vi "loadChannel.vi"(6 "xmlPath":string, 8 "error in (no error)":errorcluster, 9 "device.lvclass":refnum<class "device.lvclass">, 10 "NativeXML in":refnum<class "NativeXML.lvclass">, 11 "deviceDataBase in":refnum<class "deviceDataBase.lvclass">) -> (0 "error out":errorcluster, 1 "device.lvclass out":refnum<class "device.lvclass">, 2 "Channel.lvclass":refnum<class "Channel.lvclass">, 3 "deviceDataBase out":refnum<class "deviceDataBase.lvclass">)   [LabVIEW 2009, in "Tools.lvlib" / "DatabaseHelpers.lvlib" / "deviceDataBase.lvclass"]
uses:
  deviceDataBase.lvclass
  NativeXML/NativeXML.lvclass
  Database Objects/device/device.lvclass
  Database Objects/Channel/Channel.lvclass
  Database Objects/Channel/DigitalChannel/DigitalChannel.lvclass
  Database Objects/Channel/RfOutputChannel/RfOutputChannel.lvclass
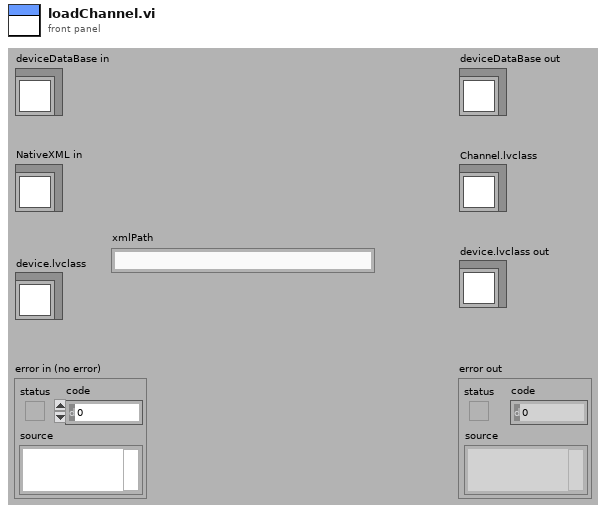
[diagram p1: front panel]
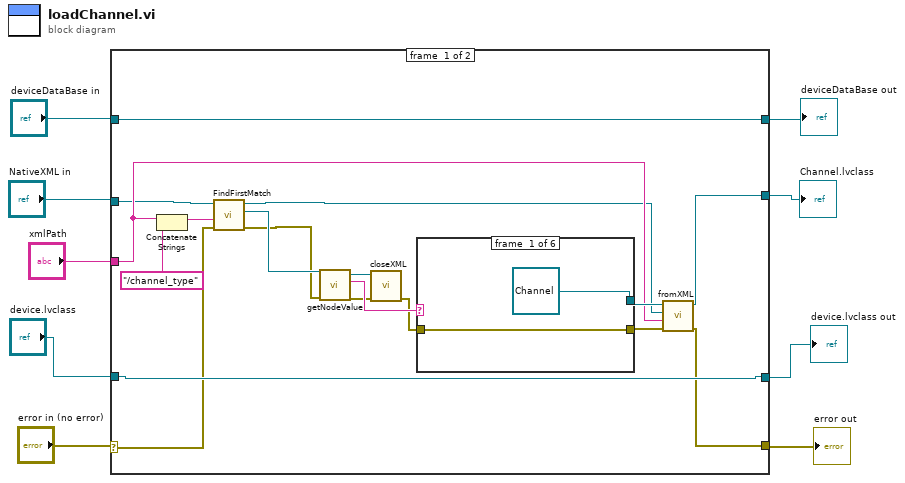
[diagram p0: block diagram]
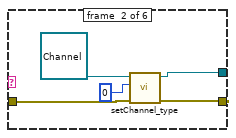
[diagram p2: hidden frame]
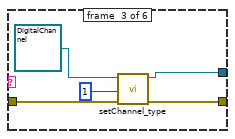
[diagram p3: hidden frame]
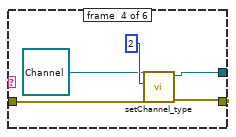
[diagram p4: hidden frame]
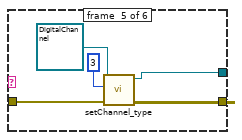
[diagram p5: hidden frame]
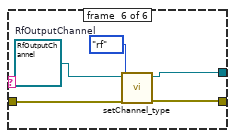
[diagram p6: hidden frame]
diagram:
  n1 = case shown="No Error" "error in (no error)" {
    selector: "error in (no error)" -> [w11 w56]
    tunnel: [w23 w56] -> w8
    tunnel: [w22 w55] -> w6
    tunnel: "deviceDataBase in" -> [w22 w55]
    tunnel: "device.lvclass" -> [w27 _]
    tunnel: "NativeXML in" -> [w14 _]
    tunnel: [w27 _] -> w3
    tunnel: [w24 _] -> w2
    tunnel: "xmlPath" -> [w17 _]
    frame #0 {
      n2 = Concatenate Strings(w17, "/channel_type") -> (w10:string)
      n3 = call "FindFirstMatch.vi"("error in (no error)"=w11, "xPath"=w10, "NativeXML in"=w14) -> ("error out"=w12:errorcluster, "NativeXML match"=w13:refnum<class "NativeXML.lvclass">, "NativeXML out"=w15:refnum<class "NativeXML.lvclass">)  [unwired: 6 in]
      n4 = call "getNodeValue.vi"("error in (no error)"=w12, "NativeXML in"=w13) -> ("error out"=w19:errorcluster, "Value"=w21:string, "NativeXML out"=w20:refnum<class "NativeXML.lvclass">)  [unwired: 7 in]
      n5 = call "closeXML.vi"("error in (no error)"=w19, "NativeXML in"=w20) -> ("error out"=w18:errorcluster)  [unwired: 9 in]
      n6 = case shown="Default" w21 {
        tunnel: w18 -> [w29 w33 w38 w42 w48 w53]
        tunnel: [w29 w32 w35 w43 w47 w51] -> w26
        tunnel: [refnum<class "Channel.lvclass"> refnum ("Tools.lvlib:DatabaseHelpers.lvlib:Channel.lvclass") w30 w36 w40 w45 w50] -> w25
        frame #0 {
        }
        frame #1 {
          n7 = call "setChannel_type.vi"("error in (no error)"=w33, "channel_type"=0, "Channel.lvclass in"=refnum<class "Channel.lvclass"> refnum ("Tools.lvlib:DatabaseHelpers.lvlib:Channel.lvclass")) -> ("error out"=w32:errorcluster, "Channel.lvclass out"=w30:refnum<class "Channel.lvclass">)  [unwired: 7 in]
        }
        frame #2 {
          n8 = call "setChannel_type.vi"("error in (no error)"=w38, "channel_type"=1, "Channel.lvclass in"=refnum<class "DigitalChannel.lvclass"> refnum ("Tools.lvlib:DatabaseHelpers.lvlib:DigitalChannel.lvclass")) -> ("error out"=w35:errorcluster, "Channel.lvclass out"=w36:refnum<class "DigitalChannel.lvclass">)  [unwired: 7 in]
        }
        frame #3 {
          n9 = call "setChannel_type.vi"("error in (no error)"=w42, "channel_type"=2, "Channel.lvclass in"=refnum<class "Channel.lvclass"> refnum ("Tools.lvlib:DatabaseHelpers.lvlib:Channel.lvclass")) -> ("error out"=w43:errorcluster, "Channel.lvclass out"=w40:refnum<class "Channel.lvclass">)  [unwired: 7 in]
        }
        frame #4 {
          n10 = call "setChannel_type.vi"("error in (no error)"=w48, "channel_type"=3, "Channel.lvclass in"=refnum<class "DigitalChannel.lvclass"> refnum ("Tools.lvlib:DatabaseHelpers.lvlib:DigitalChannel.lvclass")) -> ("error out"=w47:errorcluster, "Channel.lvclass out"=w45:refnum<class "DigitalChannel.lvclass">)  [unwired: 7 in]
        }
        frame #5 {
          w54 = refnum<class "RfOutputChannel.lvclass"> refnum  # RfOutputChannel
          n11 = call "setChannel_type.vi"("error in (no error)"=w53, "channel_type"=enum16{"ao", "do", "ai", "di", "rf"}."rf", "Channel.lvclass in"=w54) -> ("error out"=w51:errorcluster, "Channel.lvclass out"=w50:refnum<class "RfOutputChannel.lvclass">)  [unwired: 7 in]
        }
      }
      n12 = call-dynamic "fromXML.vi"("error in (no error)"=w26, "xmlPath"=w17, "channel_configXML"=w15, "Channel in"=w25) -> ("error out"=w23:errorcluster, "Channel out"=w24:refnum<class "Channel.lvclass">)  [unwired: 6 in]
    }
    frame #1 {
    }
  }
  "error out" <- w8
  "deviceDataBase out" <- w6
  "device.lvclass out" <- w3
  "Channel.lvclass" <- w2
